vi "数值控件颜色梯度.vi"() -> ()   [LabVIEW 2012]
panel:
  out "量表 4":dbl(knob) caption="颜色插值、均匀刻度" scale=0.0..100.0
  out "量表 3":dbl(knob) caption="添加刻度" scale=0.0..100.0
  out "量表 2":dbl(knob) caption="禁止颜色插值、任意刻度" scale=0.0..100.0
  out "量表":dbl(knob) caption="放置量表" scale=0.0..100.0
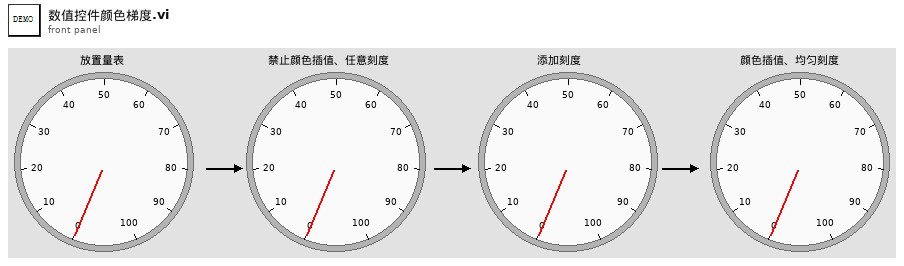
[diagram p1: front panel]
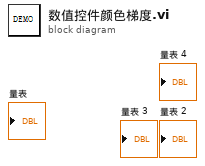
[diagram p0: block diagram]
diagram:
